vi "Status nach Timestamp einsortieren.vi"(7 "aufsteigend":bool, 8 "error in (no error)":errorcluster caption="Fehler (Eingang, kein Fehler)", 10 "GD Statuslist in":string, 11 "Statuslist old in":string="2024-03-01 Komm Error\n2024-03-01 Druck Error\n2024-03-01 Fluss Error\n2024-03-01 Komm Error\n2024-03-01 Komm Error") -> (0 "error out":errorcluster caption="Fehler (Ausgang)", 1 "merged Statuslist sorted":string, 2 "GD Statuslist out":string, 3 "Statuslist old out":string)   [LabVIEW 2020, in "Linearisierung v2.lvlib"]
uses:
  Linearisierung v2.lvlib
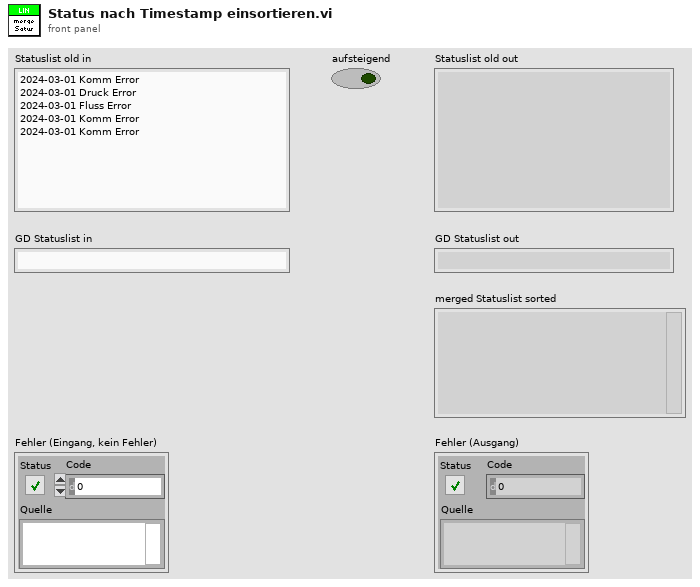
[diagram p1: front panel]
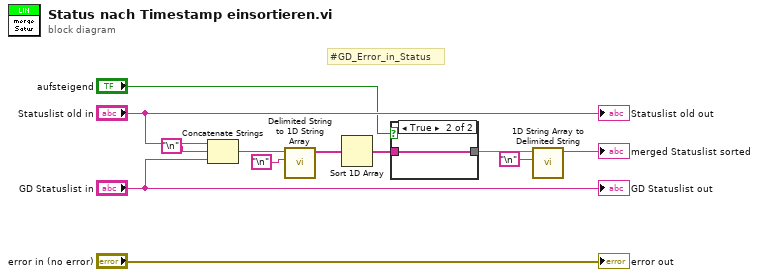
[diagram p0: block diagram]
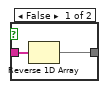
[diagram p2: hidden frame]
diagram:
  # "#GD_Error_in_Status"
  n1 = Concatenate Strings("Statuslist old in", "\n", "GD Statuslist in") -> (w7:string)
  n2 = call <vilib>:"Delimited String to 1D String Array.vi"("delimiter"="\n", "delimited string"=w7) -> ("string array"=w5:string[])  [unwired: 9 in]
  n3 = Sort 1D Array(array=w5) -> (sorted array=w3:string[])
  n4 = case shown="True" "aufsteigend" {
    tunnel: w3 -> [w14 w15]
    tunnel: [w13 w15] -> w2
    frame False {
      n5 = Reverse 1D Array(array=w14) -> (reversed array=w13:string[])
    }
    frame True {
    }
  }
  n6 = call <vilib>:"1D String Array to Delimited String.vi"("delimiter"="\n", "string array"=w2) -> ("delimited string"=→"merged Statuslist sorted":string)  [unwired: 9 in]
  "GD Statuslist out" <- "GD Statuslist in"
  "Statuslist old out" <- "Statuslist old in"
  "error out" <- "error in (no error)"
